vi "Channel Source Power Set Calibration Array.vi"(6 "Val":dbl[](array[numeric])=[0.0] format="%.2p", 8 "error in (no error)":errorcluster {"code" format="%.0x"}, 9 "PortVal":i32 format="%.0g", 10 "RepCapIdentifier":string, 11 "instrument handle":refnum<k15>) -> (0 "error out":errorcluster {"code" format="%.0x"}, 1 "ValActualSize":i32, 3 "instrument handle out":refnum<k15>)   [LabVIEW 2014, in "Agilent NA.lvlib"]
doc: "Sets the source power calibration array for the port."
uses:
  Agilent NA.lvlib
  AgNA.dll
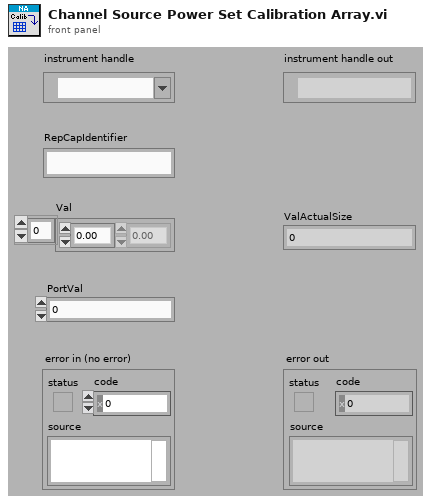
[diagram p1: front panel]
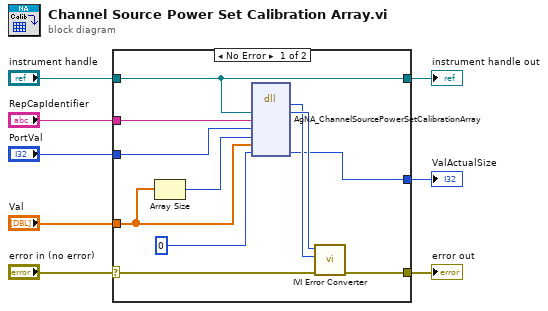
[diagram p0: block diagram]
diagram:
  n1 = case shown="No Error" "error in (no error)" {
    selector: "error in (no error)" -> [w17 w21]
    tunnel: [w16 w21] -> w8
    tunnel: "RepCapIdentifier" -> [w15 _]
    tunnel: "PortVal" -> [w14 _]
    tunnel: [w12 _] -> w4
    tunnel: "instrument handle" -> [w11 w20]
    tunnel: [w11 w20] -> w2
    tunnel: "Val" -> [w9 _]
    frame No Error {
      n2 = Array Size(array=w9) -> (size(s)=w10:i32)
      n3 = dll-call lib="AgNA**.dll" fn="AgNA_ChannelSourcePowerSetCalibrationArray"("Vi"=w11, "RepCapIdentifier"=w15, "PortVal"=w14, "ValBufferSize"=w10, "Val"=w9, "ValActualSize"=0) -> (w18:i32, "Vi"=w19:u32, "ValActualSize"=w12:i32)  [unwired: 7 in, 2 out]
      n4 = call "IVI Error Converter.vi"("error in (no error)"=w17, "IVI error code (0)"=w18, "instrument handle"=w19) -> ("error out"=w16:errorcluster)  [unwired: 7 in, 1 out]
    }
    frame Error {
    }
  }
  "error out" <- w8
  "instrument handle out" <- w2
  "ValActualSize" <- w4
